vi "Global_CMD.vi"() -> ()   [LabVIEW 2017, in "Rotation_Overlord.lvlib"]
uses:
  Rotation_Overlord.lvlib
  CLUSTER_Rotation_CMD.ctl
  ENUM_Rotation_Positon.ctl
  TypeDef/CLUSTER_Overlord_Systems.ctl
panel:
  in  "CMD_SM_Rotation":T1={"Rotation Positon"=enum."Neutral", "Enable Rotation"=TRUE, "Manual Override"=FALSE, "Arm Value"=0.0, "Claw Rotation Value"=0.0, "Lift Value"=0.0, "Enable"={"Lift"=FALSE, "Arm"=FALSE, "Claw Rotation"=FALSE}}
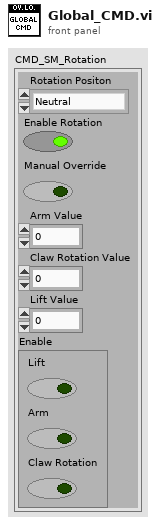
[diagram p1: front panel]
types:
  T1 = typedef "Rotation_Overlord.lvlib/CLUSTER_Rotation_CMD.ctl" = cluster{"Rotation Positon":T2, "Enable Rotation":bool, "Manual Override":bool, "Arm Value":dbl, "Claw Rotation Value":dbl, "Lift Value":dbl, "Enable":T3}
  T2 = typedef "Rotation_Overlord.lvlib/ENUM_Rotation_Positon.ctl" = enum16{"Neutral", "Pickup", "Switch", "Scale", "Climb", "Manual"}
  T3 = typedef "CLUSTER_Overlord_Systems.ctl" = cluster{"Lift":bool, "Arm":bool, "Claw Rotation":bool}
diagram:
